vi "Video.vi"() -> ()   [LabVIEW 2014]
doc: "Very simple example showing how to use the base VIs to control the AR Drone and receive and display video data."
uses:
  Global.vi
panel:
  in  "milliseconds to wait":u32=25
  in  "stop video":bool
  out "error out 3":errorcluster
  out "Video Stream 2":picture
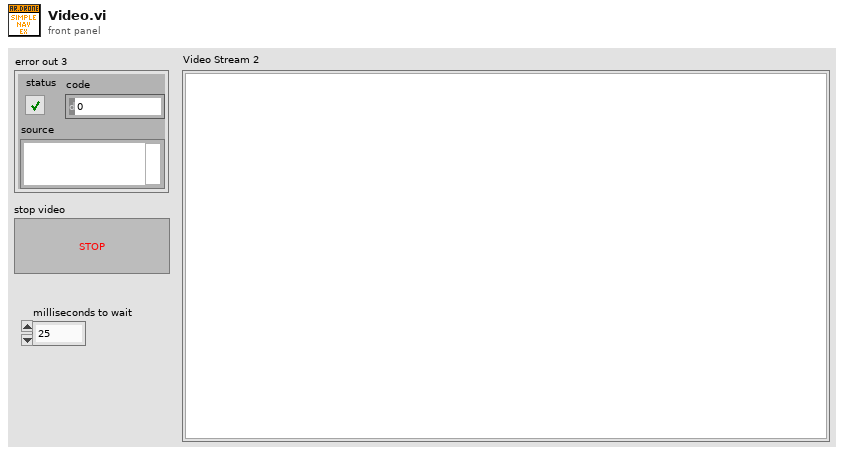
[diagram p1: front panel]
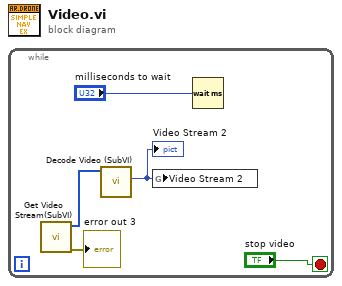
[diagram p0: block diagram]
diagram:
  n1 = while {
    stop <- "stop video" stop-if-true
    n2 = call "Get Video Stream(SubVI).vi"() -> ("error out"=→"error out 3":errorcluster, "ImgData"=w4:u8[])  [unwired: 10 in]
    n3 = call "Decode Video (SubVI).vi"("ImgData"=w4) -> ("new picture"=w3:picture)  [unwired: 9 in, 1 out]
    "Video Stream 2" <- w3
    n4 = global write "Global.vi" "Video Stream 2"(w3) -> ()
    n5 = Wait (ms)(milliseconds to wait="milliseconds to wait") -> ()  [unwired: 1 out]
  }
